vi "ReadData.vi"() -> ()   [LabVIEW 2013]
uses:
  <vilib>/Utility/file.llb/Read From Spreadsheet File (DBL).vi
  <vilib>/Analysis/NI_AALPro.lvlib
panel:
  in  "Slope (V/MHz)":dbl=0.16 format="%#_13g"
  out "Fit Error":dbl=0.00012634032702257911 format="%#_2g"
  in  "Start sigma (V)":dbl=0.01 format="%#_13g"
  in  "Start offset (V)":dbl format="%#_13g"
  in  "Start freq (MHz)":dbl=224.8 format="%#_13g"
  in  "Start amp (V)":dbl=0.25 format="%#_13g"
  out "Fit Sigma (MHz)":dbl=0.007573976601878744 format="%#_2g"
  out "Fit Freq (MHz)":dbl=224.7918158673086
  out "Fit Amplitude (V)":dbl=0.23126154565823748 format="%#_4g"
  out "NMR Graph and Fit":cluster{cluster{dbl, "Numeric":dbl}[]}[](graph)=[{[{224.59, "Numeric"=0.00012905630997347438}, {224.592, "Numeric"=0.00012905630997347438}, {224.594, "Numeric"=0.00012905630997347438}, {224.596, "Numeric"=0.00012905630997347438}, {224.598, "Numeric"=0.00012905630997347438}, {224.6, "Numeric"=0.00012905630997347438}, {224.602, "Numeric"=0.00012905630997347438}, {224.604, "Numeric"=0.00012905630997347438}, {224.606, "Numeric"=0.00012905630997347438}, {224.608, "Numeric"=0.00012905630997347438}, {224.61, "Numeric"=0.00012905630997347438}, {224.612, "Numeric"=0.00012905630997347438}, {224.614, "Numeric"=0.00012905630997347438}, {224.616, "Numeric"=0.00012905630997347438}, {224.618, "Numeric"=0.00012905630997347438}, {224.62, "Numeric"=0.00012905630997347438}, {224.622, "Numeric"=0.00012905630997347438}, {224.624, "Numeric"=0.00012905630997347438}, {224.626, "Numeric"=0.00012905630997347438}, {224.628, "Numeric"=0.00012905630997347438}, {224.63, "Numeric"=0.00012905630997347438}, {224.632, "Numeric"=0.00012905630997347438}, {224.634, "Numeric"=0.00012905630997347438}, {224.636, "Numeric"=0.00012905630997347438}, {224.638, "Numeric"=0.00012905630997347438}, {224.64, "Numeric"=0.00012905630997347438}, {224.642, "Numeric"=0.00012905630997347438}, {224.644, "Numeric"=0.00012905630997347438}, {224.646, "Numeric"=0.00012905630997347438}, {224.648, "Numeric"=0.00012905630997347438}, {224.65, "Numeric"=0.00012905630997347438}, {224.652, "Numeric"=0.00012905630997347438}, {224.654, "Numeric"=0.00012905630997347438}, {224.656, "Numeric"=0.00012905630997347438}, {224.658, "Numeric"=0.00012905630997347438}, {224.66, "Numeric"=0.00012905630997347438}, {224.662, "Numeric"=0.00012905630997347438}, {224.664, "Numeric"=0.00012905630997347438}, {224.666, "Numeric"=0.00012905630997347438}, {224.668, "Numeric"=0.00012905630997347438}, {224.67, "Numeric"=0.00012905630997347438}, {224.672, "Numeric"=0.00012905630997347438}, {224.674, "Numeric"=0.00012905630997347438}, {224.676, "Numeric"=0.00012905630997347438}, {224.678, "Numeric"=0.00012905630997347438}, {224.68, "Numeric"=0.00012905630997347438}, {224.682, "Numeric"=0.00012905630997347438}, {224.684, "Numeric"=0.00012905630997347438}, {224.686, "Numeric"=0.00012905630997347438}, {224.688, "Numeric"=0.00012905630997347438}, {224.69, "Numeric"=0.00012905630997347438}, {224.692, "Numeric"=0.00012905630997347438}, {224.694, "Numeric"=0.00012905630997347438}, {224.696, "Numeric"=0.00012905630997347438}, {224.698, "Numeric"=0.00012905630997347438}, {224.7, "Numeric"=0.00012905630997347438}, {224.702, "Numeric"=0.00012905630997347438}, {224.704, "Numeric"=0.00012905630997347438}, {224.706, "Numeric"=0.00012905630997347438}, {224.708, "Numeric"=0.00012905630997347438}, {224.71, "Numeric"=0.00012905630997347438}, {224.712, "Numeric"=0.00012905630997347438}, {224.714, "Numeric"=0.00012905630997347438}, {224.716, "Numeric"=0.00012905630997347438}, {224.718, "Numeric"=0.00012905630997347438}, {224.72, "Numeric"=0.00012905630997347438}, {224.722, "Numeric"=0.00012905630997347447}, {224.724, "Numeric"=0.00012905630997347528}, {224.726, "Numeric"=0.00012905630997348365}, {224.728, "Numeric"=0.00012905630997356318}, {224.73, "Numeric"=0.0001290563099742678}, {224.732, "Numeric"=0.00012905630998008655}, {224.734, "Numeric"=0.00012905631002486692}, {224.736, "Numeric"=0.00012905631034601408}, {224.738, "Numeric"=0.0001290563124920919}, {224.74, "Numeric"=0.00012905632585415256}, {224.742, "Numeric"=0.0001290564033618989}, {224.744, "Numeric"=0.00012905682216716945}, {224.746, "Numeric"=0.00012905892992093714}, {224.748, "Numeric"=0.00012906880876753022}, {224.75, "Numeric"=0.00012911192098785773}, {224.752, "Numeric"=0.00012928707537553243}, {224.754, "Numeric"=0.00012994940516695665}, {224.756, "Numeric"=0.00013227991617328674}, {224.758, "Numeric"=0.00013990815012219785}, {224.76, "Numeric"=0.00016312708152114446}, {224.762, "Numeric"=0.00022882119911107584}, {224.764, "Numeric"=0.0004015087208706472}, {224.766, "Numeric"=0.0008229944559368078}, {224.768, "Numeric"=0.0017774769463310537}, {224.77, "Numeric"=0.0037810708610302355}, {224.772, "Numeric"=0.007675009919288314}, {224.774, "Numeric"=0.014670681207357126}, {224.776, "Numeric"=0.02626444237735972}, {224.778, "Numeric"=0.04393792891271347}, {224.78, "Numeric"=0.06861672913378185}, {224.782, "Numeric"=0.09998637877891724}, {224.784, "Numeric"=0.13591805930188203}, {224.786, "Numeric"=0.17234226454489368}, {224.788, "Numeric"=0.2038264585795067}, {224.79, "Numeric"=0.22483869360918946}, {224.792, "Numeric"=0.23132227012385795}, {224.794, "Numeric"=0.22197201089974908}, {224.796, "Numeric"=0.19866236225506617}, {224.798, "Numeric"=0.1658350751635973}, {224.8, "Numeric"=0.1291203407931095}, {224.802, "Numeric"=0.09377729780284412}, {224.804, "Numeric"=0.06353880925735708}, {224.806, "Numeric"=0.04017233878094518}, {224.808, "Numeric"=0.023713218642755333}, {224.81, "Numeric"=0.013083787786558825}, {224.812, "Numeric"=0.006765777153416616}, {224.814, "Numeric"=0.0033000535267236806}, {224.816, "Numeric"=0.0015420992069171621}, {224.818, "Numeric"=0.000716318454786918}, {224.82, "Numeric"=0.000356684393913587}, {224.822, "Numeric"=0.00021134437566959615}, {224.824, "Numeric"=0.00015680005214654114}, {224.826, "Numeric"=0.00013778020439821732}, {224.828, "Numeric"=0.0001316147364313163}, {224.83, "Numeric"=0.00012975607567058533}, {224.832, "Numeric"=0.0001292348146244225}, {224.834, "Numeric"=0.00012909877814846118}, {224.836, "Numeric"=0.00012906573309593935}, {224.838, "Numeric"=0.00012905826001225227}, {224.84, "Numeric"=0.0001290566863381327}, {224.842, "Numeric"=0.00012905637772071298}, {224.844, "Numeric"=0.0001290563213469064}, {224.846, "Numeric"=0.00012905631175424775}, {224.848, "Numeric"=0.00012905631023351605}, {224.85, "Numeric"=0.00012905631000888996}, {224.852, "Numeric"=0.00012905630997797285}, {224.854, "Numeric"=0.0001290563099740073}, {224.856, "Numeric"=0.00012905630997353326}, {224.858, "Numeric"=0.00012905630997348046}, {224.86, "Numeric"=0.00012905630997347498}, {224.862, "Numeric"=0.00012905630997347444}, {224.864, "Numeric"=0.00012905630997347438}, {224.866, "Numeric"=0.00012905630997347438}, {224.868, "Numeric"=0.00012905630997347438}, {224.87, "Numeric"=0.00012905630997347438}, {224.872, "Numeric"=0.00012905630997347438}, {224.874, "Numeric"=0.00012905630997347438}, {224.876, "Numeric"=0.00012905630997347438}, {224.878, "Numeric"=0.00012905630997347438}, {224.88, "Numeric"=0.00012905630997347438}, {224.882, "Numeric"=0.00012905630997347438}, {224.884, "Numeric"=0.00012905630997347438}, {224.886, "Numeric"=0.00012905630997347438}, {224.888, "Numeric"=0.00012905630997347438}, {224.89, "Numeric"=0.00012905630997347438}, {224.892, "Numeric"=0.00012905630997347438}, {224.894, "Numeric"=0.00012905630997347438}, {224.896, "Numeric"=0.00012905630997347438}, {224.898, "Numeric"=0.00012905630997347438}, {224.9, "Numeric"=0.00012905630997347438}, {224.902, "Numeric"=0.00012905630997347438}, {224.904, "Numeric"=0.00012905630997347438}, {224.906, "Numeric"=0.00012905630997347438}, {224.908, "Numeric"=0.00012905630997347438}, {224.91, "Numeric"=0.00012905630997347438}, {224.912, "Numeric"=0.00012905630997347438}, {224.914, "Numeric"=0.00012905630997347438}, {224.916, "Numeric"=0.00012905630997347438}, {224.918, "Numeric"=0.00012905630997347438}, {224.92, "Numeric"=0.00012905630997347438}, {224.922, "Numeric"=0.00012905630997347438}, {224.924, "Numeric"=0.00012905630997347438}, {224.926, "Numeric"=0.00012905630997347438}, {224.928, "Numeric"=0.00012905630997347438}, {224.93, "Numeric"=0.00012905630997347438}, {224.932, "Numeric"=0.00012905630997347438}, {224.934, "Numeric"=0.00012905630997347438}, {224.936, "Numeric"=0.00012905630997347438}, {224.938, "Numeric"=0.00012905630997347438}, {224.94, "Numeric"=0.00012905630997347438}, {224.942, "Numeric"=0.00012905630997347438}, {224.944, "Numeric"=0.00012905630997347438}, {224.946, "Numeric"=0.00012905630997347438}, {224.948, "Numeric"=0.00012905630997347438}, {224.95, "Numeric"=0.00012905630997347438}, {224.952, "Numeric"=0.00012905630997347438}, {224.954, "Numeric"=0.00012905630997347438}, {224.956, "Numeric"=0.00012905630997347438}, {224.958, "Numeric"=0.00012905630997347438}, {224.96, "Numeric"=0.00012905630997347438}, {224.962, "Numeric"=0.00012905630997347438}, {224.964, "Numeric"=0.00012905630997347438}, {224.966, "Numeric"=0.00012905630997347438}, {224.968, "Numeric"=0.00012905630997347438}, {224.97, "Numeric"=0.00012905630997347438}, {224.972, "Numeric"=0.00012905630997347438}, {224.974, "Numeric"=0.00012905630997347438}, {224.976, "Numeric"=0.00012905630997347438}, {224.978, "Numeric"=0.00012905630997347438}, {224.98, "Numeric"=0.00012905630997347438}, {224.982, "Numeric"=0.00012905630997347438}, {224.984, "Numeric"=0.00012905630997347438}, {224.986, "Numeric"=0.00012905630997347438}, {224.988, "Numeric"=0.00012905630997347438}, {224.99, "Numeric"=0.00012905630997347438}]}, {[{224.59, "Numeric"=-0.007907899999997275}, {224.592, "Numeric"=0.0042641000000012}, {224.594, "Numeric"=0.0002640000000042192}, {224.596, "Numeric"=0.00011150000000269278}, {224.598, "Numeric"=0.005722900000001165}, {224.6, "Numeric"=-0.007706299999995819}, {224.602, "Numeric"=-0.016714399999997343}, {224.604, "Numeric"=0.008874600000001131}, {224.606, "Numeric"=-0.00811229999999585}, {224.608, "Numeric"=-0.01218179999999738}, {224.61, "Numeric"=0.007566800000001091}, {224.612, "Numeric"=-0.006568999999995884}, {224.614, "Numeric"=-0.004869999999997415}, {224.616, "Numeric"=-0.0018258999999989436}, {224.618, "Numeric"=0.006957700000004077}, {224.62, "Numeric"=-0.0014804999999974526}, {224.622, "Numeric"=-0.019389099999998983}, {224.624, "Numeric"=-0.00403129999999596}, {224.626, "Numeric"=0.001636500000002511}, {224.628, "Numeric"=-0.006719399999999015}, {224.63, "Numeric"=0.002590600000004002}, {224.632, "Numeric"=0.007545000000002473}, {224.634, "Numeric"=-0.006028699999999054}, {224.636, "Numeric"=-0.011433499999996037}, {224.638, "Numeric"=-0.0021143999999975634}, {224.64, "Numeric"=0.01074700000000091}, {224.642, "Numeric"=0.01090310000000393}, {224.644, "Numeric"=0.006215400000002404}, {224.646, "Numeric"=-0.00915119999999913}, {224.648, "Numeric"=-0.013346099999996103}, {224.65, "Numeric"=-0.0026583999999976356}, {224.652, "Numeric"=-0.0028081999999991607}, {224.654, "Numeric"=-0.019972399999996147}, {224.656, "Numeric"=-0.014746499999997675}, {224.658, "Numeric"=-0.0259002999999992}, {224.66, "Numeric"=-0.02092619999999618}, {224.662, "Numeric"=-0.00617209999999771}, {224.664, "Numeric"=-0.010043599999999236}, {224.666, "Numeric"=-0.000558299999996216}, {224.668, "Numeric"=-0.010553199999997747}, {224.67, "Numeric"=0.011924860000000728}, {224.672, "Numeric"=0.014837360000003748}, {224.674, "Numeric"=0.007364000000002221}, {224.676, "Numeric"=0.002810300000000694}, {224.678, "Numeric"=0.01029506000000371}, {224.68, "Numeric"=-0.005911699999997817}, {224.682, "Numeric"=0.011929130000000655}, {224.684, "Numeric"=0.0006585000000036735}, {224.686, "Numeric"=0.005662200000002147}, {224.688, "Numeric"=0.002330700000000619}, {224.69, "Numeric"=0.01805663000000364}, {224.692, "Numeric"=0.014986049000002109}, {224.694, "Numeric"=-0.0028649999999994184}, {224.696, "Numeric"=0.005104150000003603}, {224.698, "Numeric"=0.015748890000002073}, {224.7, "Numeric"=0.004337800000000546}, {224.702, "Numeric"=0.005441210000003565}, {224.704, "Numeric"=0.021866710000002038}, {224.706, "Numeric"=0.01755474000000051}, {224.708, "Numeric"=0.00916790000000353}, {224.71, "Numeric"=0.012917123000002001}, {224.712, "Numeric"=0.005767750000000473}, {224.714, "Numeric"=0.008081100000003493}, {224.716, "Numeric"=0.0078088400000019655}, {224.718, "Numeric"=-0.005180899999999565}, {224.72, "Numeric"=-0.002152699999996545}, {224.722, "Numeric"=-0.002711099999998072}, {224.724, "Numeric"=-0.00042299999999959904}, {224.726, "Numeric"=0.00933813500000342}, {224.728, "Numeric"=0.002512150000001893}, {224.73, "Numeric"=-0.010610399999999636}, {224.732, "Numeric"=0.006970050000003383}, {224.734, "Numeric"=-0.004145999999998144}, {224.736, "Numeric"=-0.0004525899999996714}, {224.738, "Numeric"=-0.013614799999996654}, {224.74, "Numeric"=0.00059335000000182}, {224.742, "Numeric"=0.0012418100000002917}, {224.744, "Numeric"=-0.006017599999996689}, {224.746, "Numeric"=-0.019890999999998216}, {224.748, "Numeric"=-0.008932899999999747}, {224.75, "Numeric"=-0.011436999999996724}, {224.752, "Numeric"=-0.007322599999998254}, {224.754, "Numeric"=-0.014192199999999782}, {224.756, "Numeric"=0.0002661600000032384}, {224.758, "Numeric"=0.00323997000000171}, {224.76, "Numeric"=-0.012448499999999817}, {224.762, "Numeric"=0.004470290000003202}, {224.764, "Numeric"=-0.0006545399999983263}, {224.766, "Numeric"=-0.011648699999999854}, {224.768, "Numeric"=0.006741780000003165}, {224.77, "Numeric"=0.0023562050000016373}, {224.772, "Numeric"=0.021325000000000108}, {224.774, "Numeric"=0.02757630000000313}, {224.776, "Numeric"=0.0331829000000016}, {224.778, "Numeric"=0.04570090000000007}, {224.78, "Numeric"=0.04948100000000309}, {224.782, "Numeric"=0.09449880000000156}, {224.784, "Numeric"=0.11224800000000003}, {224.786, "Numeric"=0.17086900000000305}, {224.788, "Numeric"=0.20964400000000155}, {224.79, "Numeric"=0.24206100000000455}, {224.792, "Numeric"=0.26774200000000303}, {224.794, "Numeric"=0.22720200000000149}, {224.796, "Numeric"=0.1760930000000045}, {224.798, "Numeric"=0.137047000000003}, {224.8, "Numeric"=0.10349600000000145}, {224.802, "Numeric"=0.08939360000000447}, {224.804, "Numeric"=0.07260780000000296}, {224.806, "Numeric"=0.06554110000000142}, {224.808, "Numeric"=0.06757080000000443}, {224.81, "Numeric"=0.028172200000002912}, {224.812, "Numeric"=0.037250000000001386}, {224.814, "Numeric"=0.025749000000004404}, {224.816, "Numeric"=0.018888900000002873}, {224.818, "Numeric"=0.020881200000001345}, {224.82, "Numeric"=0.0014036700000043655}, {224.822, "Numeric"=0.003937650000002838}, {224.824, "Numeric"=0.00918390000000131}, {224.826, "Numeric"=0.01415160000000433}, {224.828, "Numeric"=0.013189000000002803}, {224.83, "Numeric"=0.0016574000000012723}, {224.832, "Numeric"=0.01277210000000429}, {224.834, "Numeric"=0.003796300000002765}, {224.836, "Numeric"=0.006370700000001237}, {224.838, "Numeric"=-0.002112299999995744}, {224.84, "Numeric"=-0.005868849999997271}, {224.842, "Numeric"=-0.0220986999999988}, {224.844, "Numeric"=-0.012459599999995779}, {224.846, "Numeric"=-0.01601400999999731}, {224.848, "Numeric"=-0.000877179999998836}, {224.85, "Numeric"=-0.005794219999995817}, {224.852, "Numeric"=-0.0032016699999973443}, {224.854, "Numeric"=-0.006600479999998873}, {224.856, "Numeric"=-0.008910599999995852}, {224.858, "Numeric"=-0.011596849999997381}, {224.86, "Numeric"=0.0023452000000010916}, {224.862, "Numeric"=-0.00807580999999589}, {224.864, "Numeric"=-0.004383159999997417}, {224.866, "Numeric"=-0.012419188999998946}, {224.868, "Numeric"=-0.009661929999995924}, {224.87, "Numeric"=-0.0021293999999974535}, {224.872, "Numeric"=0.013010300000001017}, {224.874, "Numeric"=-0.0010712999999959623}, {224.876, "Numeric"=-0.01728686999999749}, {224.878, "Numeric"=-0.01914467999999902}, {224.88, "Numeric"=0.0035969000000040004}, {224.882, "Numeric"=-0.006447229999997526}, {224.884, "Numeric"=0.00042980000000094644}, {224.886, "Numeric"=-0.008547799999996036}, {224.888, "Numeric"=-0.0077697199999975635}, {224.89, "Numeric"=-0.0029731999999990915}, {224.892, "Numeric"=-0.005779499999996071}, {224.894, "Numeric"=-0.0028949999999975974}, {224.896, "Numeric"=0.01575110000000087}, {224.898, "Numeric"=0.015136800000003895}, {224.9, "Numeric"=-0.004029999999997634}, {224.902, "Numeric"=0.01701550000000084}, {224.904, "Numeric"=0.010084800000003856}, {224.906, "Numeric"=0.0045479000000023286}, {224.908, "Numeric"=0.011635400000000802}, {224.91, "Numeric"=0.006335000000003817}, {224.912, "Numeric"=-0.01165841999999771}, {224.914, "Numeric"=-0.0015855999999992362}, {224.916, "Numeric"=-0.005939199999996215}, {224.918, "Numeric"=0.006140100000002254}, {224.92, "Numeric"=0.002853100000000726}, {224.922, "Numeric"=0.011677700000003746}, {224.924, "Numeric"=-0.002835299999997782}, {224.926, "Numeric"=0.000952400000000693}, {224.928, "Numeric"=-0.00692759999999629}, {224.93, "Numeric"=-0.002244299999997819}, {224.932, "Numeric"=-0.0019531999999993464}, {224.934, "Numeric"=-0.010265799999996328}, {224.936, "Numeric"=-0.010128899999997854}, {224.938, "Numeric"=-0.014005759999999381}, {224.94, "Numeric"=0.01838670000000364}, {224.942, "Numeric"=-0.013195599999997892}, {224.944, "Numeric"=-0.00690939999999942}, {224.946, "Numeric"=0.000892700000003601}, {224.948, "Numeric"=0.011846500000002074}, {224.95, "Numeric"=0.005029200000000542}, {224.952, "Numeric"=0.003182400000003565}, {224.954, "Numeric"=0.002961400000002036}, {224.956, "Numeric"=-0.006192799999999492}, {224.958, "Numeric"=0.008886200000003525}, {224.96, "Numeric"=-0.0018504999999979996}, {224.962, "Numeric"=0.0012824000000004714}, {224.964, "Numeric"=-0.0017225999999965075}, {224.966, "Numeric"=0.003648700000001965}, {224.968, "Numeric"=0.010340600000000432}, {224.97, "Numeric"=0.0036071000000034575}, {224.972, "Numeric"=-0.003807799999998071}, {224.974, "Numeric"=-0.0073872999999996004}, {224.976, "Numeric"=-0.00221219999999658}, {224.978, "Numeric"=0.0022329000000018903}, {224.98, "Numeric"=0.009817400000000365}, {224.982, "Numeric"=0.0033050000000033816}, {224.984, "Numeric"=-0.003400399999998145}, {224.986, "Numeric"=0.00301910000000033}, {224.988, "Numeric"=-0.009846299999996654}, {224.99, "Numeric"=0.0016314000000018161}]}]
  out "File size (bytes)":i32=3882
  out "Waveform Array":dbl[][](array[numeric])=[[224.59, -0.0399079], [224.592, -0.0274159], [224.594, -0.031096], [224.596, -0.0309285], [224.598, -0.0249971], [224.6, -0.0381063], [224.602, -0.0467944], [224.604, -0.0208854], [224.606, -0.0375523], [224.608, -0.0413018], [224.61, -0.0212332], [224.612, -0.035049], [224.614, -0.03303], [224.616, -0.0296659], [224.618, -0.0205623], [224.62, -0.0286805], [224.622, -0.0462691], [224.624, -0.0305913], [224.626, -0.0246035], [224.628, -0.0326394], [224.63, -0.0230094], [224.632, -0.017735], [224.634, -0.0309887], [224.636, -0.0360735], [224.638, -0.0264344], [224.64, -0.013253], [224.642, -0.0127769], [224.644, -0.0171446], [224.646, -0.0321912], [224.648, -0.0360661], [224.65, -0.0250584], [224.652, -0.0248882], [224.654, -0.0417324], [224.656, -0.0361865], [224.658, -0.0470203], [224.66, -0.0417262], [224.662, -0.0266521], [224.664, -0.0302036], [224.666, -0.0203983], [224.668, -0.0300732], [224.67, -0.00727514], [224.672, -0.00404264], [224.674, -0.011196], [224.676, -0.0154297], [224.678, -0.00762494], [224.68, -0.0235117], [224.682, -0.00535087], [224.684, -0.0163015], [224.686, -0.0109778], [224.688, -0.0139893], [224.69, 0.00205663], [224.692, -0.000693951], [224.694, -0.018225], [224.696, -0.00993585], [224.698, 0.00102889], [224.7, -0.0100622], [224.702, -0.00863879], [224.704, 0.00810671], [224.706, 0.00411474], [224.708, -0.0039521], [224.71, 0.000117123], [224.712, -0.00671225], [224.714, -0.0040789], [224.716, -0.00403116], [224.718, -0.0167009], [224.72, -0.0133527], [224.722, -0.0135911], [224.724, -0.010983], [224.726, -0.000901865], [224.728, -0.00740785], [224.73, -0.0202104], [224.732, -0.00230995], [224.734, -0.013106], [224.736, -0.00909259], [224.738, -0.0219348], [224.74, -0.00740665], [224.742, -0.00643819], [224.744, -0.0133776], [224.746, -0.026931], [224.748, -0.0156529], [224.75, -0.017837], [224.752, -0.0134026], [224.754, -0.0199522], [224.756, -0.00517384], [224.758, -0.00188003], [224.76, -0.0172485], [224.762, -9.71e-06], [224.764, -0.00481454], [224.766, -0.0154887], [224.768, 0.00322178], [224.77, -0.000843795], [224.772, 0.018445], [224.774, 0.0250163], [224.776, 0.0309429], [224.778, 0.0437809], [224.78, 0.047881], [224.782, 0.0932188], [224.784, 0.111288], [224.786, 0.170229], [224.788, 0.209324], [224.79, 0.242061], [224.792, 0.268062], [224.794, 0.227842], [224.796, 0.177053], [224.798, 0.138327], [224.8, 0.105096], [224.802, 0.0913136], [224.804, 0.0748478], [224.806, 0.0681011], [224.808, 0.0704508], [224.81, 0.0313722], [224.812, 0.04077], [224.814, 0.029589], [224.816, 0.0230489], [224.818, 0.0253612], [224.82, 0.00620367], [224.822, 0.00905765], [224.824, 0.0146239], [224.826, 0.0199116], [224.828, 0.019269], [224.83, 0.0080574], [224.832, 0.0194921], [224.834, 0.0108363], [224.836, 0.0137307], [224.838, 0.0055677], [224.84, 0.00213115], [224.842, -0.0137787], [224.844, -0.0038196], [224.846, -0.00705401], [224.848, 0.00840282], [224.85, 0.00380578], [224.852, 0.00671833], [224.854, 0.00363952], [224.856, 0.0016494], [224.858, -0.00071685], [224.86, 0.0135452], [224.862, 0.00344419], [224.864, 0.00745684], [224.866, -0.000259189], [224.868, 0.00281807], [224.87, 0.0106706], [224.872, 0.0261303], [224.874, 0.0123687], [224.876, -0.00352687], [224.878, -0.00506468], [224.88, 0.0179969], [224.882, 0.00827277], [224.884, 0.0154698], [224.886, 0.0068122], [224.888, 0.00791028], [224.89, 0.0130268], [224.892, 0.0105405], [224.894, 0.013745], [224.896, 0.0327111], [224.898, 0.0324168], [224.9, 0.01357], [224.902, 0.0349355], [224.904, 0.0283248], [224.906, 0.0231079], [224.908, 0.0305154], [224.91, 0.025535], [224.912, 0.00786158], [224.914, 0.0182544], [224.916, 0.0142208], [224.918, 0.0266201], [224.92, 0.0236531], [224.922, 0.0327977], [224.924, 0.0186047], [224.926, 0.0227124], [224.928, 0.0151524], [224.93, 0.0201557], [224.932, 0.0207668], [224.934, 0.0127742], [224.936, 0.0132311], [224.938, 0.00967424], [224.94, 0.0423867], [224.942, 0.0111244], [224.944, 0.0177306], [224.946, 0.0258527], [224.948, 0.0371265], [224.95, 0.0306292], [224.952, 0.0291024], [224.954, 0.0292014], [224.956, 0.0203672], [224.958, 0.0357662], [224.96, 0.0253495], [224.962, 0.0288024], [224.964, 0.0261174], [224.966, 0.0318087], [224.968, 0.0388206], [224.97, 0.0324071], [224.972, 0.0253122], [224.974, 0.0220527], [224.976, 0.0275478], [224.978, 0.0323129], [224.98, 0.0402174], [224.982, 0.034025], [224.984, 0.0276396], [224.986, 0.0343791], [224.988, 0.0218337], [224.99, 0.0336314]]
  out "File name":string="C:\\Documents and Settings\\Patrick McGaughey\\Desktop\\rssmt\\wfm.txt"
  # "Saves data to spreadsheet file"
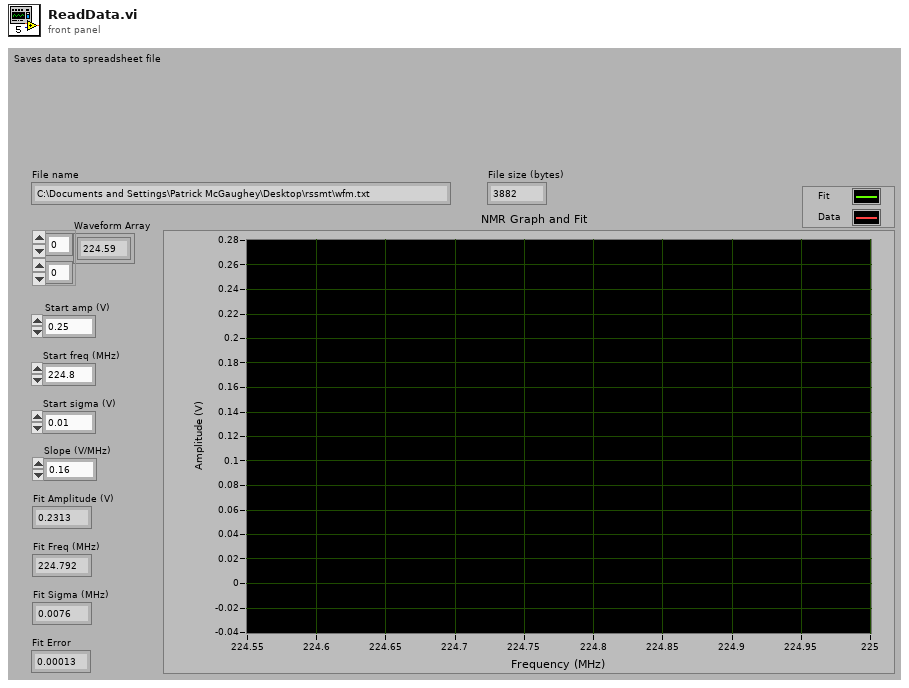
[diagram p1: front panel]
types:
  T1 = cluster{"Start amp (V)":dbl, "Start freq (MHz)":dbl, "Start sigma (V)":dbl, "Start offset (V)":dbl}
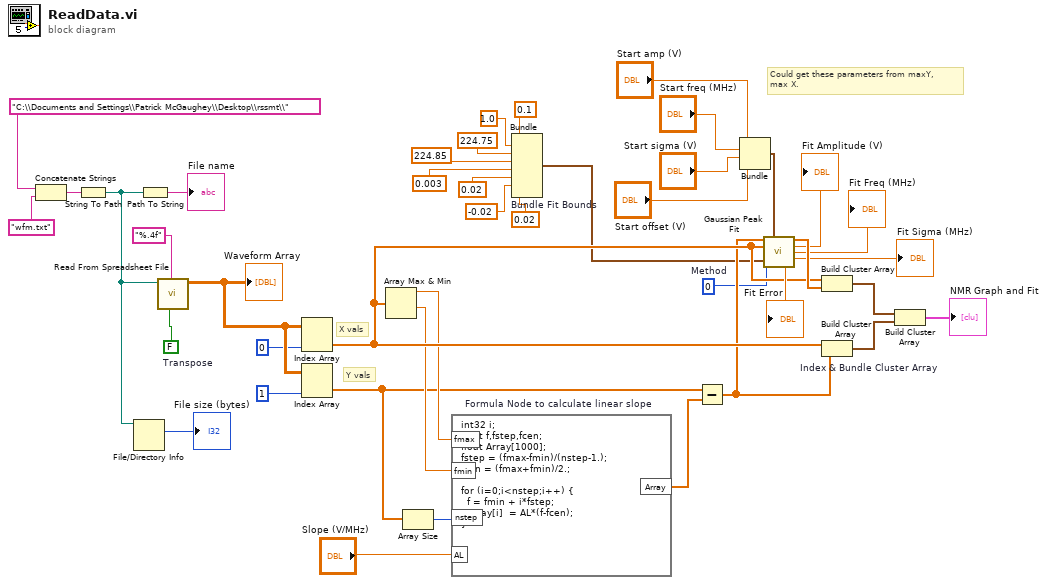
[diagram p0: block diagram]
diagram:
  w1 = 0  # Method
  w38 = FALSE  # Transpose
  # "Could get these parameters from maxY,\nmax X."
  # "Y vals"
  # "X vals"
  n1 = Concatenate Strings "Concatenate Strings"("C:\\Documents and Settings\\Patrick McGaughey\\Desktop\\rssmt\\", "wfm.txt") -> (w41:string)
  n2 = String To Path(string=w41) -> (path=w37:path)
  n3 = File/Directory Info(path=w37) -> (size=→"File size (bytes)":i64)  [unwired: 1 in, 6 out]
  n4 = Path To String(path=w37) -> (string=→"File name":string)
  n5 = call-poly <vilib>:"Read From Spreadsheet File.vi"("transpose (no:F)"=w38, "format (%.3f)"="%.4f", "file path (dialog if empty)"=w37) -> ("all rows"=w35:dbl[][])  [unwired: 4 in, 4 out]
  "Waveform Array" <- w35
  n6 = Index Array "Index Array"(array=w35, index (col)=0) -> (element=w17:dbl[])  [unwired: 1 in]
  n7 = Index Array(array=w35, index (col)=1) -> (element=w12:dbl[])  [unwired: 1 in]
  n8 = Array Max & Min(array=w17) -> (max value=w15:dbl, min value=w16:dbl)  [unwired: 2 out]
  n9 = Array Size(array=w12) -> (size(s)=w18:i32)
  n10 = formula code="int32 i;\nfloat f,fstep,fcen;\nfloat Array[1000];\nfstep = (fmax-fmin)/(nstep-1.);\nfcen = (fmax+fmin)/2.;\n\nfor (i=0;i<nstep;i++) {\n  f = fmin + i*fstep;\n  Array[i]  = AL*(f-fcen);\n}" "Formula Node to calculate linear slope"("nstep"=w18, "fmin"=w16, "fmax"=w15, "AL"="Slope (V/MHz)") -> ("Array"=w13:dbl[])
  n11 = Bundle "Bundle Fit Bounds"(0.1, 1.0, 224.75, 224.85, 0.003, 0.02, -0.02, 0.02) -> (w2:cluster{dbl, dbl, dbl, dbl, dbl, dbl, dbl, dbl})  [unwired: 1 in]
  n12 = Subtract(x=w12, y=w13) -> (x-y=w11:dbl[])
  n13 = Bundle "Bundle"("Start amp (V)"="Start amp (V)", "Start freq (MHz)"="Start freq (MHz)", "Start sigma (V)"="Start sigma (V)", "Start offset (V)"="Start offset (V)") -> (w27:T1)  [unwired: 1 in]
  n14 = call <vilib>:"Gaussian Peak Fit.vi"("Y"=w11, "initial guess"=w27, "X"=w17, "method"=w1, "parameter bounds"=w2) -> ("Best Gaussian Fit"=w32:dbl[], "amplitude"=→"Fit Amplitude (V)":dbl, "center"=→"Fit Freq (MHz)":dbl, "standard deviation"=→"Fit Sigma (MHz)":dbl, "residue"=→"Fit Error":dbl)  [unwired: 4 in, 2 out]
  n15 = Build Cluster Array ("Index & Bundle Cluster Array")(w17, w32) -> (w26:cluster{dbl, "Numeric":dbl}[])
  n16 = Build Cluster Array "Index & Bundle Cluster Array"(w17, w11) -> (w25:cluster{dbl, dbl}[])
  n17 = Build Cluster Array "Build Cluster Array"(w26, w25) -> (→"NMR Graph and Fit":cluster{cluster{dbl, "Numeric":dbl}[]}[])
